vi "Read stopped event.vi"(8 "error in (no error)":errorcluster, 11 "ConfigurableActor in":refnum<class "ConfigurableActor.lvclass">) -> (0 "error out":errorcluster, 2 "stopped event":refnum<user-event>, 3 "ConfigurableActor out":refnum<class "ConfigurableActor.lvclass">)   [LabVIEW 2014, in "ConfigurableActor.lvclass"]
uses:
  ConfigurableActor.lvclass
  ConfigurableActor.lvclass/ConfigurableActor.ctl
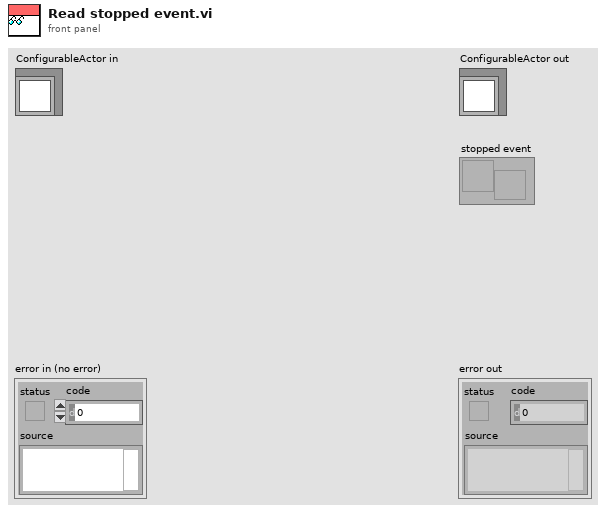
[diagram p1: front panel]
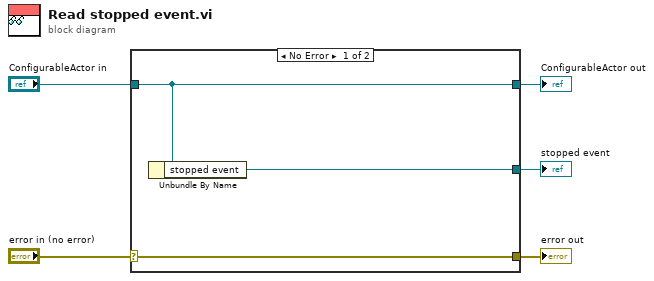
[diagram p0: block diagram]
diagram:
  n1 = case shown="No Error" "error in (no error)" {
    selector: "error in (no error)" -> [w8 w9]
    tunnel: [w8 w9] -> w4
    tunnel: [w7 w10] -> w2
    tunnel: "ConfigurableActor in" -> [w7 w10]
    tunnel: [w6 _] -> w1
    frame No Error {
      n2 = Unbundle By Name(w7) -> ("stopped event"=w6:refnum<user-event>)
    }
    frame Error {
    }
  }
  "error out" <- w4
  "ConfigurableActor out" <- w2
  "stopped event" <- w1
